vi "data sample half(50ms).vi"(8 "Number of Remove data":i32, 11 "배열":string[](array[string])) -> (3 "배열 2":string[](array[string]))   [LabVIEW 2015]
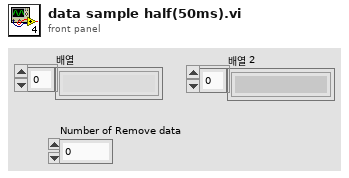
[diagram p1: front panel]
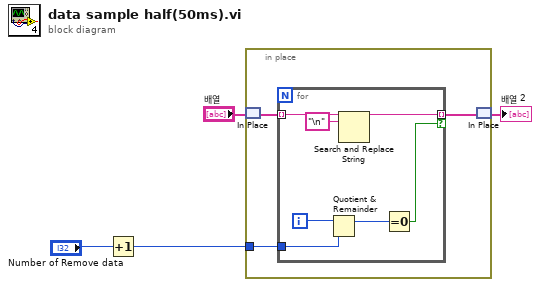
[diagram p0: block diagram]
diagram:
  n1 = Increment(x="Number of Remove data") -> (x+1=w1:i32)
  n2 = in-place {
    in-place-border: w1 -> [w5]
    n3 = in-place-match #1("배열") -> (w7:string[])
    n4 = for {
      tunnel: w7 -> [w11] mode=indexing
      tunnel: [w9] -> w6 mode=indexing if=w12
      tunnel: w5 -> [w8]
      i -> [w14]
      n5 = Quotient & Remainder(x=w14, y=w8) -> (x-y*floor(x/y)=w13:i32)  [unwired: 1 out]
      n6 = Search and Replace String(input string=w11, search string="\n" ("검색 문자열")) -> (result string=w9:string)  [unwired: 6 in, 3 out]
      n7 = Equal To 0?(x=w13) -> (x = 0?=w12:bool)
    }
    n8 = in-place-match #1(w6) -> (→"배열 2":string[])
  }
